vi "Write JSON Setup to CCD.vi"(8 "error in (no error)":errorcluster, 11 "Interface in":refnum<class "Interface.lvclass">) -> (0 "error out":errorcluster, 3 "Interface out":refnum<class "Interface.lvclass">)   [LabVIEW 2018, in "Interface.lvclass"]
uses:
  Interface.lvclass
  Interface.lvclass/Interface.ctl
  CCD/CCD.lvclass
panel:
  in  "Camera Setup":T1={"Image Name"="Image", "# Images"=0, "Exposure Time"=0.0, "Pre-amp gain"=0, "Readout Rate"=0, "EM Mode"=0, "EM Gain"=2, "Vertical Binning"=1, "Horizontal Binning"=1, "Initial Line"=1, "Initial Cloumn"=1, "Final Line"=1024, "Final Column"=1024, "Kinetic Serie Length"=0, "Image path"="", "Shutter Mode"=2} {"Shutter Mode" items=["Auto", "Open", "Closed"]; "EM Mode" items=["Electron Multiplying", "Conventional"]; "Readout Rate" items=["1 MHz", "10 MHz", "20 MHz", "30 MHz"]; "Pre-amp gain" items=["Gain 1", "Gain 2"]}
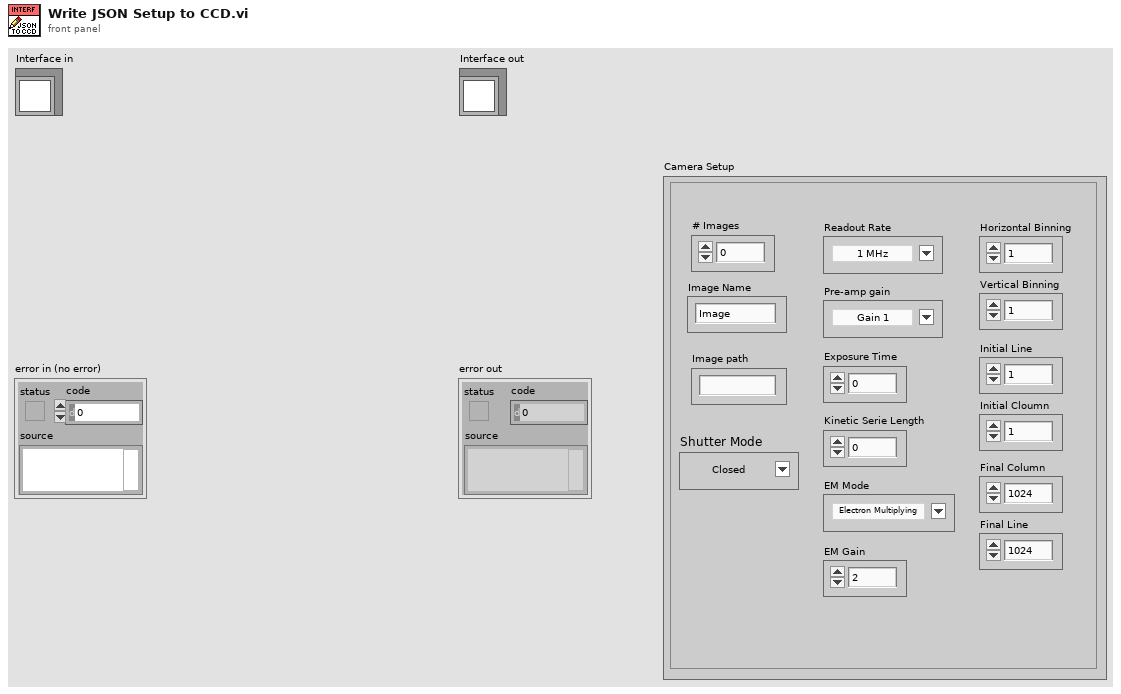
[diagram p1: front panel]
types:
  T1 = cluster{"Image Name":string, "# Images":u32, "Exposure Time":dbl, "Pre-amp gain":u8, "Readout Rate":u8, "EM Mode":u8, "EM Gain":u16, "Vertical Binning":u16, "Horizontal Binning":u16, "Initial Line":u16, "Initial Cloumn":u16, "Final Line":u16, "Final Column":u16, "Kinetic Serie Length":u32, "Image path":string, "Shutter Mode":u16}
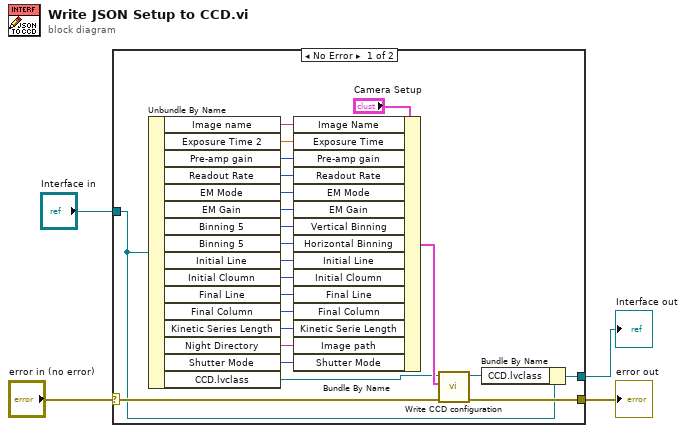
[diagram p0: block diagram]
diagram:
  n1 = case shown="No Error" "error in (no error)" {
    selector: "error in (no error)" -> [w23 w29]
    tunnel: [w22 w29] -> w3
    tunnel: [w10 w28] -> w1
    tunnel: "Interface in" -> [w11 w28]
    frame No Error {
      n2 = Unbundle By Name(w11) -> ("Image name"=w5:string, "Exposure Time 2"=w27:dbl, "Pre-amp gain"=w21:u8, "Readout Rate"=w20:u8, "EM Mode"=w19:u8, "EM Gain"=w18:u32, "Binning 5"=w17:u8, "Binning 5"=w16:u8, "Initial Line"=w15:u16, "Initial Cloumn"=w14:u16, "Final Line"=w13:u16, "Final Column"=w12:u16, "Kinetic Series Length"=w26:u16, "Night Directory"=w8:string, "Shutter Mode"=w7:u16, "CCD.lvclass"=w9:refnum<class "CCD.lvclass">)
      n3 = Bundle By Name(cluster="Camera Setup", "Image Name"=w5, "Exposure Time"=w27, "Pre-amp gain"=w21, "Readout Rate"=w20, "EM Mode"=w19, "EM Gain"=w18, "Vertical Binning"=w17, "Horizontal Binning"=w16, "Initial Line"=w15, "Initial Cloumn"=w14, "Final Line"=w13, "Final Column"=w12, "Kinetic Serie Length"=w26, "Image path"=w8, "Shutter Mode"=w7) -> (w25:T1)
      n4 = call "Write CCD configuration.vi"("error in (no error)"=w23, "Camera Setup"=w25, "CCD in"=w9) -> ("error out"=w22:errorcluster, "CCD out"=w24:refnum<class "CCD.lvclass">)  [unwired: 7 in]
      n5 = Bundle By Name(cluster=w11, "CCD.lvclass"=w24) -> (w10:refnum<class "Interface.lvclass">)
    }
    frame Error {
    }
  }
  "error out" <- w3
  "Interface out" <- w1
